vi "grow_pops.vi"(0 "rho+ array":dbl[](array[numeric]), 1 "rho0 array":dbl[](array[numeric]), 2 "Sat pol in":dbl, 3 "Zero Ensemble Condition":dbl[](array[numeric]), 4 "rho- array":dbl[](array[numeric]), 5 "rho+ condition":dbl[](array[numeric]), 6 "Microwave power":dbl, 7 "rho0 condition":dbl[](array[numeric]), 8 "Microwave on":bool, 9 "Zero Ensemble Array":dbl[](array[numeric]), 10 "Zero Level Power":dbl, 12 "Decay rate":dbl, 13 "rho- condition":dbl[](array[numeric])) -> (14 "rho+ array out":dbl[](array[numeric]), 15 "rho0 array out":dbl[](array[numeric]), 17 "rho0 decay out":dbl[](array[numeric]), 18 "rho- array out":dbl[](array[numeric]), 19 "Zero Ensemble Out":dbl[](array[numeric]))   [LabVIEW 2018]
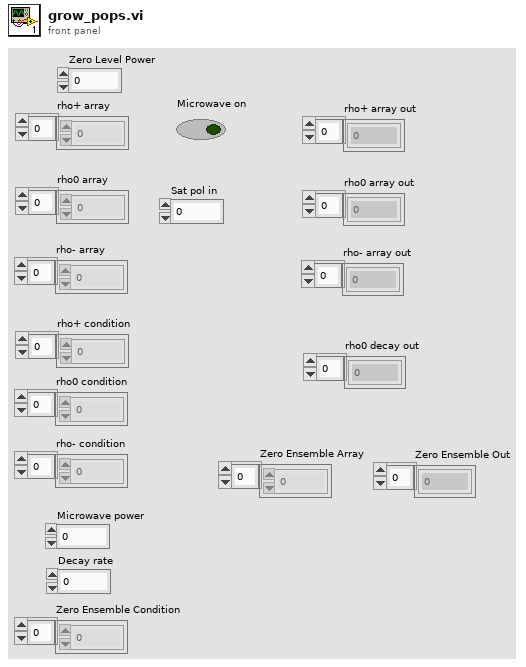
[diagram p1: front panel]
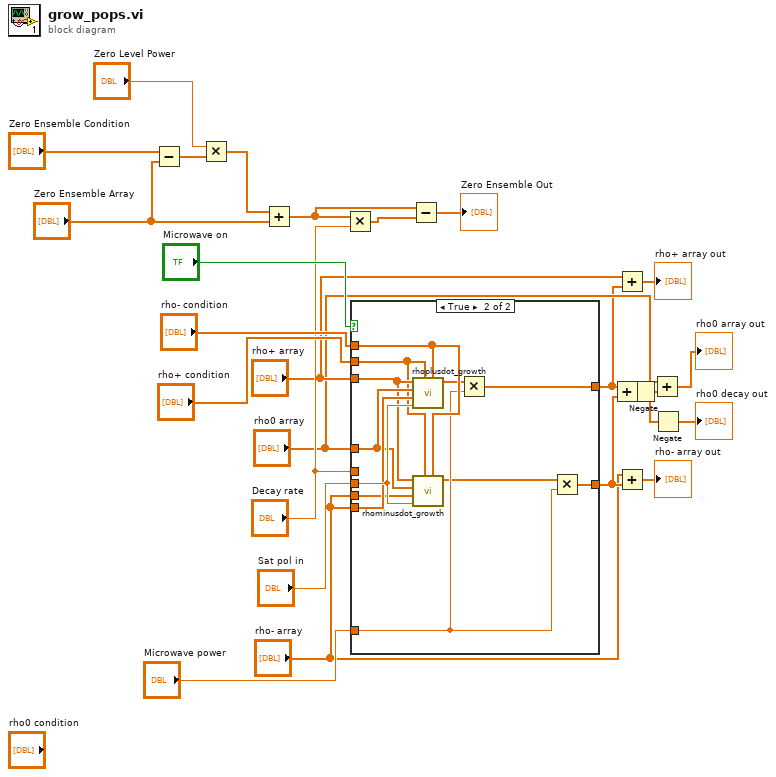
[diagram p0: block diagram]
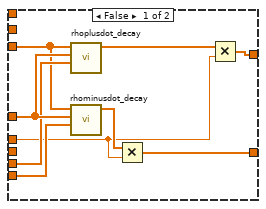
[diagram p2: hidden frame]
diagram:
  n1 = Subtract(x="Zero Ensemble Condition", y="Zero Ensemble Array") -> (x-y=w23:dbl[])
  n2 = Multiply(x="Zero Level Power", y=w23) -> (x*y=w22:dbl[])
  n3 = Add(x=w22, y="Zero Ensemble Array") -> (x+y=w19:dbl[])
  n4 = Multiply(x=w19, y="Decay rate") -> (x*y=w20:dbl[])
  n5 = case shown="True" "Microwave on" {
    tunnel: "Sat pol in" -> [_ w46]
    tunnel: "rho- condition" -> [_ w40]
    tunnel: "rho- array" -> [w34 w45]
    tunnel: "rho0 array" -> [w33 w44]
    tunnel: "rho+ condition" -> [_ w41]
    tunnel: "rho+ array" -> [w31 w42]
    tunnel: "rho- array" -> [w32 w43]
    tunnel: "Microwave power" -> [_ w38]
    tunnel: "Decay rate" -> [w28 _]
    tunnel: [w27 w36] -> w9
    tunnel: [w26 w35] -> w8
    frame False {
      n6 = call "rhoplusdot_decay.vi"("rho- in"=w32, "rho0 in"=w33, "rho+ in"=w31) -> ("rho+ dot out"=w29:dbl[])  [unwired: 8 in]
      n7 = call "rhominusdot_decay.vi"("rho- in"=w34, "rho0 in"=w33, "rho+ in"=w31) -> ("rho+ dot out"=w30:dbl[])  [unwired: 8 in]
      n8 = Multiply(x=w30, y=w28) -> (x*y=w26:dbl[])
      n9 = Multiply(x=w29, y=w28) -> (x*y=w27:dbl[])
    }
    frame True {
      n10 = call "rhoplusdot_growth.vi"("rho- sat in"=w40, "rho+ sat in"=w41, "Sat pol in"=w46, "rho- in"=w45, "rho0 in"=w44, "rho+ in"=w42) -> ("rho+ dot out"=w39:dbl[])  [unwired: 5 in]
      n11 = call "rhominusdot_growth.vi"("rho- sat in"=w40, "rho+ sat in"=w41, "Sat pol in"=w46, "rho- in"=w43, "rho0 in"=w44, "rho+ in"=w42) -> ("rho- dot out"=w37:dbl[])  [unwired: 5 in]
      n12 = Multiply(x=w39, y=w38) -> (x*y=w36:dbl[])
      n13 = Multiply(x=w37, y=w38) -> (x*y=w35:dbl[])
    }
  }
  n14 = Subtract(x=w19, y=w20) -> (x-y=→"Zero Ensemble Out":dbl[])
  n15 = Add(x=w9, y=w8) -> (x+y=w3:dbl[])
  n16 = Add(x="rho+ array", y=w9) -> (x+y=→"rho+ array out":dbl[])
  n17 = Add(x="rho- array", y=w8) -> (x+y=→"rho- array out":dbl[])
  n18 = Negate(x=w3) -> (-x=w1:dbl[])
  n19 = Add(x="rho0 array", y=w1) -> (x+y=→"rho0 array out":dbl[])
  n20 = Negate(x=w1) -> (-x=→"rho0 decay out":dbl[])
